vi "Receiver_Statistics.vi"(8 "error in (no error)":errorcluster, 9 "Frame ID":u32, 10 "Node ID":u32, 11 "Initialize ?":bool) -> (0 "error out":errorcluster, 2 "Output":T1, 3 "Received Packet Data":T1[](array[typedef]))   [LabVIEW 2017]
uses:
  Controls/ADCP_UI/ADCP_UI_Data_Packet_Receiver_Parameters.ctl
panel:
  out "Execution time (ms)":u32
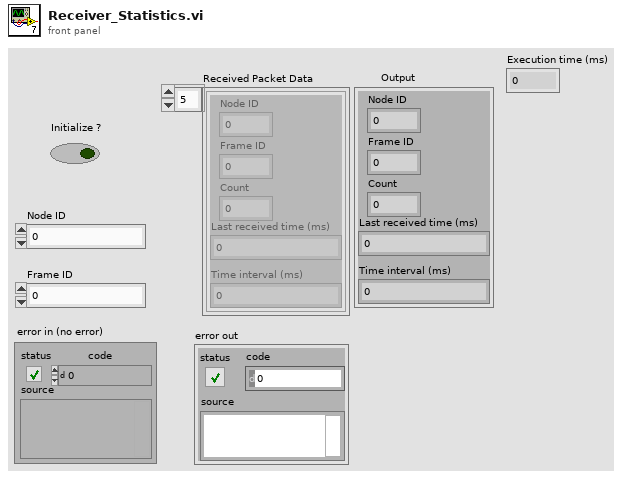
[diagram p1: front panel]
types:
  T1 = typedef "ADCP_UI_Data_Packet_Receiver_Parameters.ctl" = cluster{"Node ID":u32, "Frame ID":u32, "Count":u32, "Last received time (ms)":u32, "Time interval (ms)":u32}
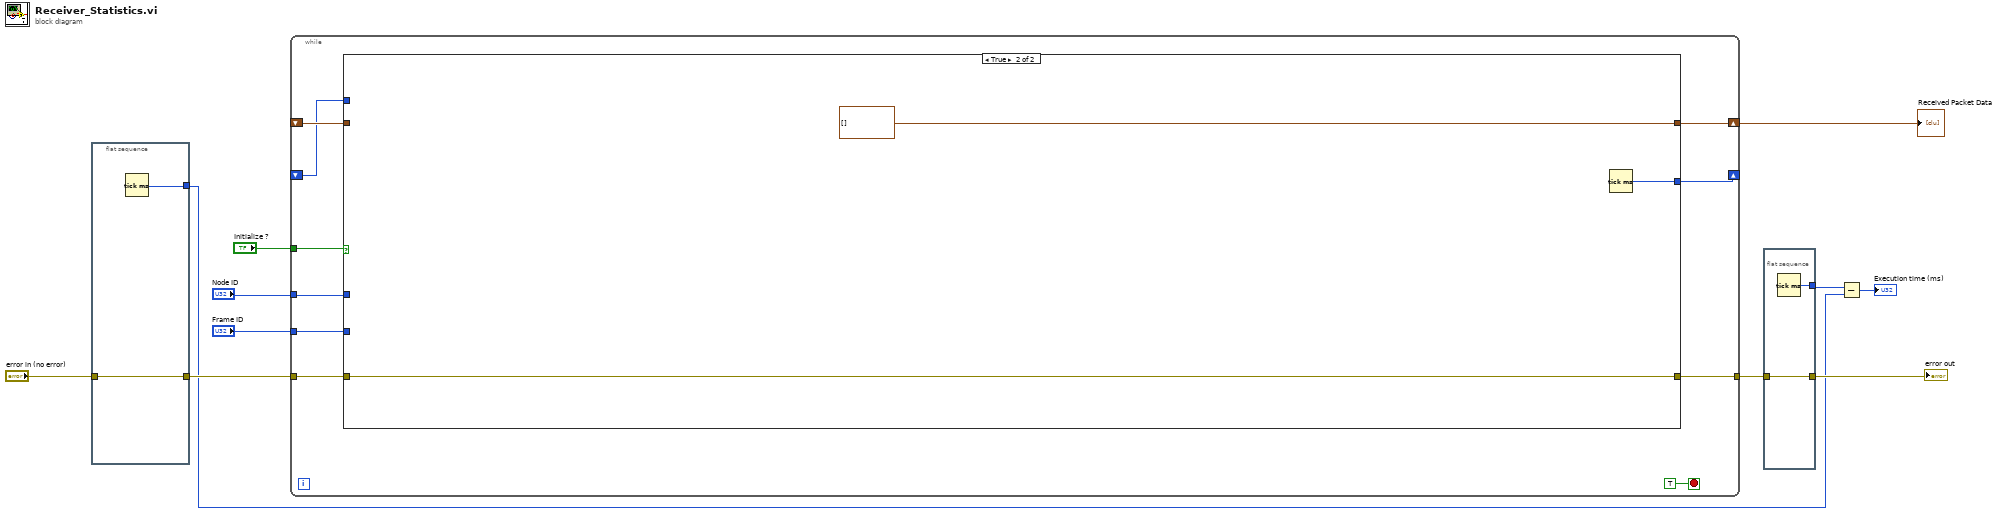
[diagram p0: block diagram]
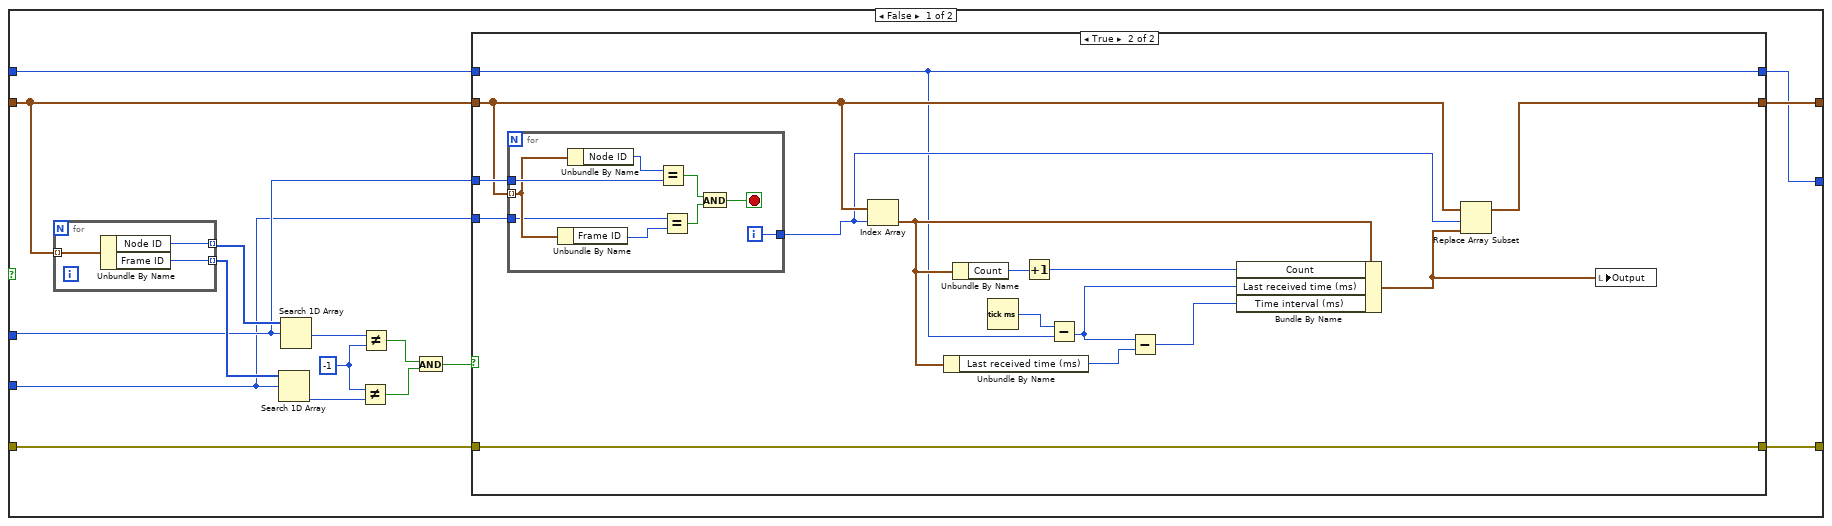
[diagram p2: hidden frame]
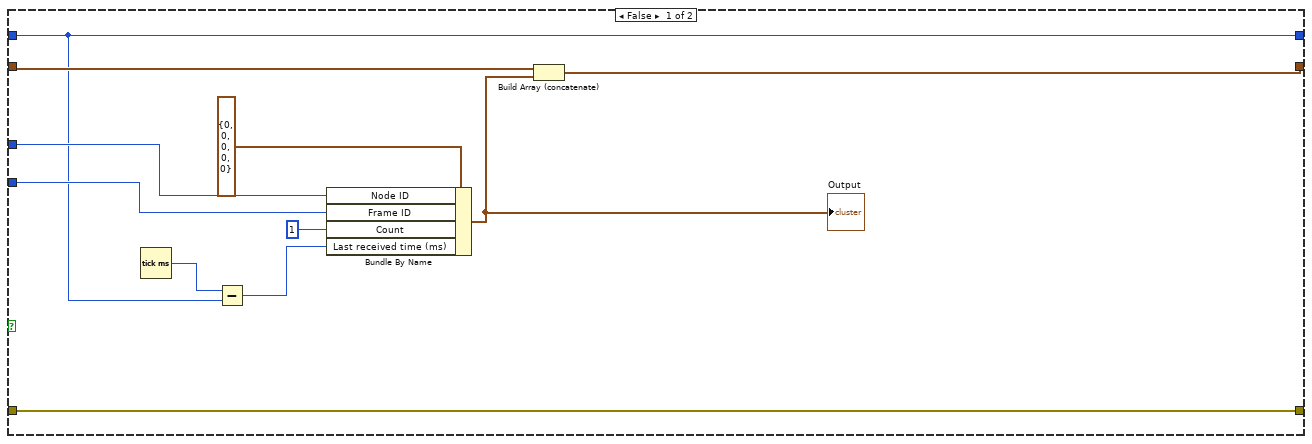
[diagram p3: hidden frame]
diagram:
  n1 = flat-sequence {
    tunnel: "error in (no error)" -> [w13]
    tunnel: [w13] -> w6
    tunnel: [w12] -> w2
    frame #0 {
      n2 = Tick Count (ms)() -> (millisecond timer value=w12:u32)
    }
  }
  n3 = while {
    tunnel: w6 -> [w22]
    tunnel: "Initialize ?" -> [w21]
    tunnel: "Node ID" -> [w20]
    tunnel: "Frame ID" -> [w19]
    shift-right: [w18] -> w8
    shift-left: _ -> [w17]
    tunnel: [w16] -> w5
    shift-right: [w15] -> _
    shift-left: _ -> [w14]
    stop <- TRUE stop-if-true
    n4 = case shown="True" w21 {
      tunnel: w22 -> [w27 w79]
      tunnel: w20 -> [w30 _]
      tunnel: w19 -> [w29 _]
      tunnel: [w28 T1[] []] -> w18
      tunnel: w17 -> [w31 _]
      tunnel: [w26 w79] -> w16
      tunnel: [w24 w78] -> w15
      tunnel: w14 -> [w25 _]
      frame False {
        w35 = -1 ("y")
        n5 = for {
          tunnel: w31 -> [w77] mode=indexing
          tunnel: [w76] -> w39 mode=indexing
          tunnel: [w75] -> w38 mode=indexing
          n6 = Unbundle By Name(w77) -> ("Node ID"=w76:u32, "Frame ID"=w75:u32)
        }
        n7 = Search 1D Array(1D array=w38, element=w29) -> (index of element=w36:i32)  [unwired: 1 in]
        n8 = Search 1D Array(1D array=w39, element=w30) -> (index of element=w37:i32)  [unwired: 1 in]
        n9 = Not Equal?(x=w35, y=w36) -> (x != y?=w33:bool)
        n10 = Not Equal?(x=w37, y=w35) -> (x != y?=w34:bool)
        n11 = And(x=w34, y=w33) -> (x .and. y?=w32:bool)
        n12 = case shown="True" w32 {
          tunnel: w31 -> [w47 w61]
          tunnel: w30 -> [w50 w65]
          tunnel: w29 -> [w49 w64]
          tunnel: [w46 w59] -> w28
          tunnel: w27 -> [w45 w58]
          tunnel: [w45 w58] -> w26
          tunnel: w25 -> [w40 w52]
          tunnel: [w40 w52] -> w24
          frame False {
            n13 = Tick Count (ms)() -> (millisecond timer value=w42:u32)
            n14 = Subtract(x=w42, y=w40) -> (x-y=w41:u32)
            n15 = Bundle By Name(cluster=T1 {"Node ID"=0, "Frame ID"=0, "Count"=0, "Last received time (ms)"=0, "Time interval (ms)"=0} ("Cluster"), "Node ID"=w50, "Frame ID"=w49, "Count"=u32 1, "Last received time (ms)"=w41) -> (w43:T1)
            "Output" <- w43
            n16 = Build Array (concatenate)(w47, w43) -> (w46:T1[])
          }
          frame True {
            n17 = for {
              tunnel: w61 -> [w72] mode=indexing
              tunnel: w65 -> [w73]
              tunnel: w64 -> [w70]
              tunnel: [w66] -> w60
              i -> [w66]
              stop <- w67 stop-if-true
              n18 = Unbundle By Name(w72) -> ("Frame ID"=w71:u32)
              n19 = Unbundle By Name(w72) -> ("Node ID"=w74:u32)
              n20 = Equal?(x=w74, y=w73) -> (x = y?=w68:bool)
              n21 = Equal?(x=w70, y=w71) -> (x = y?=w69:bool)
              n22 = And(x=w68, y=w69) -> (x .and. y?=w67:bool)
            }
            n23 = Index Array(array=w61, index=w60) -> (element=w56:T1)
            n24 = Unbundle By Name(w56) -> ("Last received time (ms)"=w55:u32)
            n25 = Unbundle By Name(w56) -> ("Count"=w63:u32)
            n26 = Tick Count (ms)() -> (millisecond timer value=w53:u32)
            n27 = Increment(x=w63) -> (x+1=w62:u32)
            n28 = Subtract(x=w53, y=w52) -> (x-y=w51:u32)
            n29 = Subtract(x=w51, y=w55) -> (x-y=w54:u32)
            n30 = Bundle By Name(cluster=w56, "Count"=w62, "Last received time (ms)"=w51, "Time interval (ms)"=w54) -> (w57:T1)
            n31 = Replace Array Subset(array=w61, new element=w57, index=w60) -> (w59:T1[])
            n32 = local write "Output"(w57) -> ()
          }
        }
      }
      frame True {
        n33 = Tick Count (ms)() -> (millisecond timer value=w78:u32)
      }
    }
  }
  "Received Packet Data" <- w8
  n34 = flat-sequence {
    tunnel: w5 -> [w82]
    tunnel: [w82] -> w4
    tunnel: [w81] -> w3
    frame #0 {
      n35 = Tick Count (ms)() -> (millisecond timer value=w81:u32)
    }
  }
  n36 = Subtract(x=w3, y=w2) -> (x-y=→"Execution time (ms)":u32)
  "error out" <- w4
